vi "hamamatsuBufferKeepAlive.vi"   [LabVIEW 2017]
uses:
  globalDevices.vi
  globalUtilities.vi
types:
  T1 = cluster{"height":i32, "width":i32, "datatype":i32}
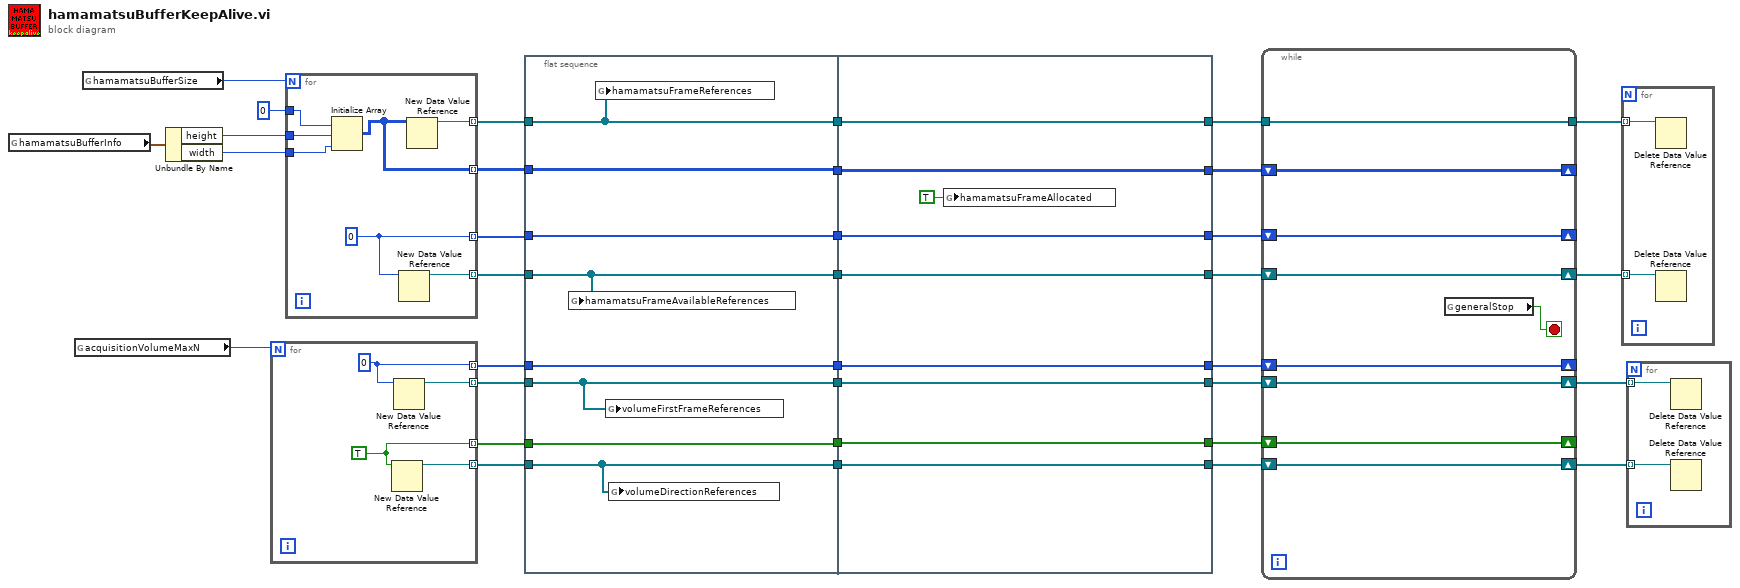
[diagram p0: block diagram]
diagram:
  n1 = global read "globalDevices.vi" "hamamatsuBufferInfo"() -> (w34:T1)
  n2 = global read "globalUtilities.vi" "acquisitionVolumeMaxN"() -> (w3:i32)
  n3 = global read "globalDevices.vi" "hamamatsuBufferSize"() -> (w23:i32)
  n4 = Unbundle By Name(w34) -> ("height"=w33:i32, "width"=w32:i32)
  n5 = for {
    N: w3 -> [_]
    tunnel: [w38] -> w14 mode=indexing
    tunnel: [w37] -> w13 mode=indexing
    tunnel: [w36] -> w4 mode=indexing
    tunnel: [w35] -> w5 mode=indexing
    w36 = TRUE
    w35 = u32 0 ("element")
    n6 = New Data Value Reference(data value=w36) -> (data value reference=w38:refnum<data-value>)  [unwired: 1 in, 1 out]
    n7 = New Data Value Reference(data value=w35) -> (data value reference=w37:refnum<data-value>)  [unwired: 1 in, 1 out]
  }
  n8 = for {
    N: w23 -> [_]
    tunnel: w33 -> [w44]
    tunnel: w32 -> [w43]
    tunnel: u16 0 -> [w45]
    tunnel: [w42] -> w30 mode=indexing
    tunnel: [w41] -> w29 mode=indexing
    tunnel: [w40] -> w8 mode=indexing
    tunnel: [w39] -> w7 mode=indexing
    w40 = 0
    n9 = Initialize Array(w45, w44, w43) -> (w41:u16[][])
    n10 = New Data Value Reference(data value=w40) -> (data value reference=w39:refnum<data-value>)  [unwired: 1 in, 1 out]
    n11 = New Data Value Reference(data value=w41) -> (data value reference=w42:refnum<data-value>)  [unwired: 1 in, 1 out]
  }
  n12 = flat-sequence {
    tunnel: w30 -> [w53]
    tunnel: w29 -> [w52]
    tunnel: [w53] -> w28
    tunnel: [w52] -> w27
    tunnel: [w51] -> w22
    tunnel: w8 -> [w51]
    tunnel: w7 -> [w50]
    tunnel: [w50] -> w20
    tunnel: w5 -> [w49]
    tunnel: [w49] -> w18
    tunnel: w4 -> [w48]
    tunnel: [w48] -> w16
    tunnel: w14 -> [w46]
    tunnel: w13 -> [w47]
    tunnel: [w47] -> w12
    tunnel: [w46] -> w10
    tunnel: [w61] -> w25
    tunnel: [w62] -> w26
    tunnel: w28 -> [w62]
    tunnel: w27 -> [w61]
    tunnel: w22 -> [w59]
    tunnel: [w59] -> w21
    tunnel: w20 -> [w58]
    tunnel: [w58] -> w19
    tunnel: w18 -> [w57]
    tunnel: [w57] -> w17
    tunnel: w16 -> [w56]
    tunnel: [w56] -> w15
    tunnel: w12 -> [w55]
    tunnel: [w55] -> w11
    tunnel: w10 -> [w54]
    tunnel: [w54] -> w9
    frame #0 {
      n13 = global write "globalDevices.vi" "hamamatsuFrameAvailableReferences"(w50) -> ()
      n14 = global write "globalDevices.vi" "hamamatsuFrameReferences"(w53) -> ()
      n15 = global write "globalUtilities.vi" "volumeFirstFrameReferences"(w47) -> ()
      n16 = global write "globalUtilities.vi" "volumeDirectionReferences"(w46) -> ()
    }
    frame #1 {
      n17 = global write "globalDevices.vi" "hamamatsuFrameAllocated"(TRUE ("hamamatsuFrameAllocated")) -> ()
    }
  }
  n18 = while {
    tunnel: w26 -> [w70]
    tunnel: [w70] -> w24
    shift-right: [w69] -> _
    shift-left: w25 -> [w69]
    shift-right: [w68] -> _
    shift-left: w21 -> [w68]
    shift-right: [w67] -> w6
    shift-left: w19 -> [w67]
    shift-right: [w66] -> _
    shift-left: w17 -> [w66]
    shift-right: [w65] -> _
    shift-left: w15 -> [w65]
    shift-right: [w64] -> w2
    shift-left: w11 -> [w64]
    shift-right: [w63] -> w1
    shift-left: w9 -> [w63]
    stop <- w71 stop-if-true
    n19 = global read "globalUtilities.vi" "generalStop"() -> (w71:bool)
  }
  n20 = for {
    tunnel: w24 -> [w73] mode=indexing
    tunnel: w6 -> [w72] mode=indexing
    n21 = Delete Data Value Reference(data value reference=w73) -> ()  [unwired: 1 in, 2 out]
    n22 = Delete Data Value Reference(data value reference=w72) -> ()  [unwired: 1 in, 2 out]
  }
  n23 = for {
    tunnel: w2 -> [w75] mode=indexing
    tunnel: w1 -> [w74] mode=indexing
    n24 = Delete Data Value Reference(data value reference=w75) -> ()  [unwired: 1 in, 2 out]
    n25 = Delete Data Value Reference(data value reference=w74) -> ()  [unwired: 1 in, 2 out]
  }
